vi "Build Diagnostics Engine Group.vi"(8 "error in (no error)":errorcluster, 11 "Section Ref in":T1 format="%.0x") -> (0 "error out":errorcluster, 2 "Group":T2 {"VS Refs" format="%.0x"}, 3 "Section Ref out":T1 format="%.0x")   [LabVIEW 2017, in "NI 272x Resistive Simulation Custom Device Configuration.lvlib"]
uses:
  NI 272x Resistive Simulation Custom Device Configuration.lvlib
  <vilib>/NI Veristand/Custom Device API/Custom Device Item Ref.ctl
  <vilib>/NI Veristand/Custom Device Tools/Custom Device Utility Library/NI VeriStand - Search for Item by Name.vi
  Globals/Names.vi
  <vilib>/NI VeriStand/Custom Device Tools/Custom Device Utility Library/Custom Device Utility Library.lvlib
  <vilib>/NI VeriStand/Custom Device API/Custom Device API.lvlib
  NI 272x Resistive Simulation Custom Device Shared.lvlib
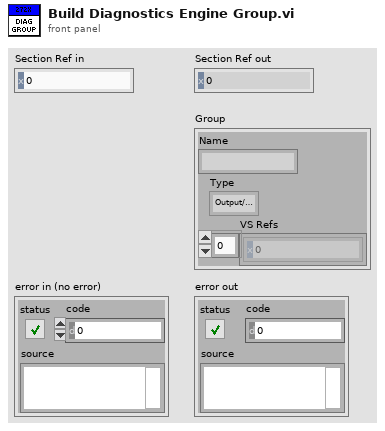
[diagram p1: front panel]
types:
  T1 = typedef "Custom Device API.lvlib/Custom Device Item Ref.ctl" = u64
  T2 = cluster{"Name":string, "Type":enum16{"Output/Write", "Input/Read", "Input/ReadWrite"}, "VS Refs":T1[]}
  T3 = enum16{"Output/Write", "Input/Read", "Input/ReadWrite"}
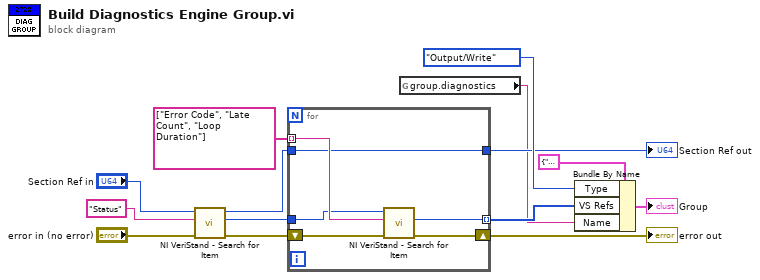
[diagram p0: block diagram]
diagram:
  n1 = call-poly <vilib>:"NI VeriStand - Search for Item.vi"("error in"="error in (no error)", "Item Name"="Status", "Section Ref in"="Section Ref in") -> ("error out"=w5:errorcluster, "Item Ref"=w6:T1, "Section Ref out"=w7:T1)  [unwired: 5 in, 1 out]
  n2 = for {
    tunnel: string[] ["Error Code", "Late Count", "Loop Duration"] -> [w20] mode=indexing
    tunnel: w6 -> [w18]
    shift-right: [w17] -> w8
    shift-left: w5 -> [w19]
    tunnel: w7 -> [w16]
    tunnel: [w16] -> w9
    tunnel: [w15] -> w12 mode=indexing
    n3 = call-poly <vilib>:"NI VeriStand - Search for Item.vi"("error in"=w19, "Item Name"=w20, "Section Ref in"=w18) -> ("error out"=w17:errorcluster, "Item Ref"=w15:T1)  [unwired: 5 in, 2 out]
  }
  "Section Ref out" <- w9
  "error out" <- w8
  n4 = global read "Names.vi" "group.diagnostics"() -> (w1:string)
  n5 = Bundle By Name(cluster=T2 {"Name"="", "Type"=enum."Output/Write", "VS Refs"=[]} ("Group"), "Type"=T3."Output/Write", "VS Refs"=w12, "Name"=w1) -> (→"Group":T2)
